vi "GUI Panel.vi"(8 "error in (no error)":errorcluster) -> (0 "error out":errorcluster)   [LabVIEW 2015]
uses:
  Button_UI/Private/Button_UI(Classic).ctl
  Button_UI/Button_UI.lvclass
panel:
  in  "Temparate":T1
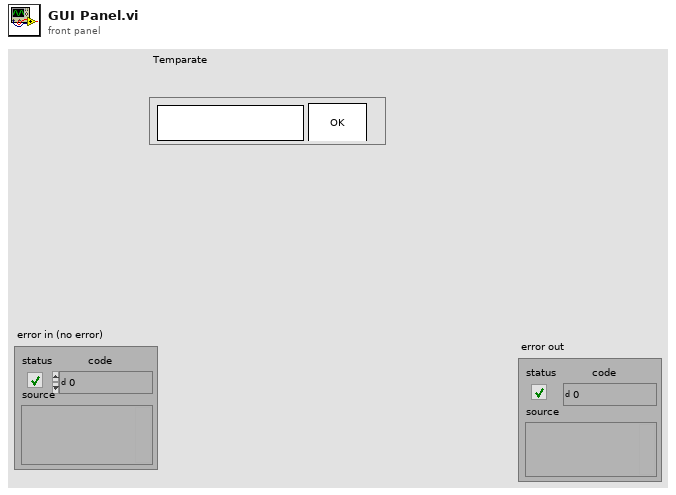
[diagram p1: front panel]
types:
  T1 = typedef "Button_UI.lvclass/Button_UI(Classic).ctl" = cluster{"Protocol":string, "Push":bool}
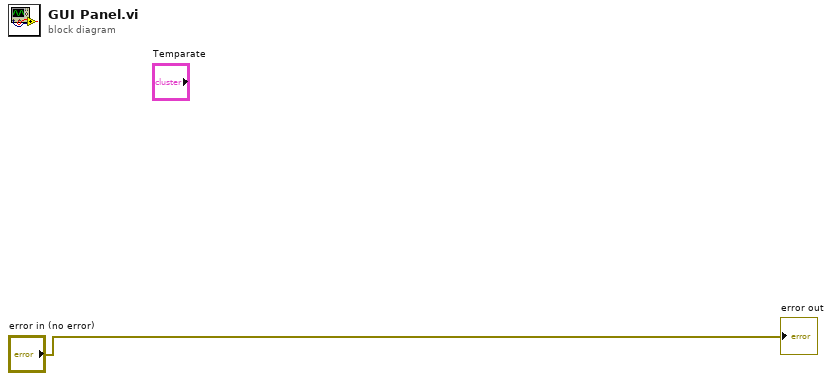
[diagram p0: block diagram]
diagram:
  "error out" <- "error in (no error)"
